vi "Order control references by label order.vi"(8 "error in":errorcluster, 10 "Ordered Labels":string[](array[string]), 11 "Control References":refnum<vi>[](array[refnum])) -> (0 "error out":errorcluster, 3 "Ordered control references":refnum<vi>[](array[refnum]))   [LabVIEW 2017, in "verticalDistribution.lvlib"]
doc: "For a given list of control references, this VI orders the references according to the label array.\n\nEach label that doesn't have a matching control reference is assigned a Not a Refnum value."
uses:
  <vilib>/Utility/vertDist/verticalDistribution.lvlib
panel:
  # "Each label that doesn't \nhave a matching control\nreference will be assigned\na Not a Refnum value."
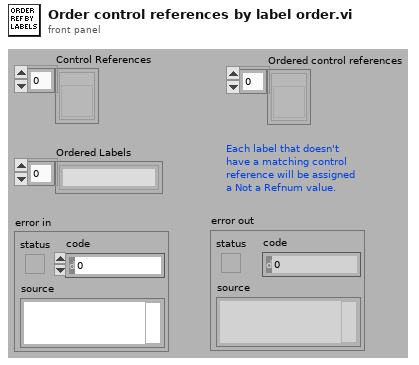
[diagram p1: front panel]
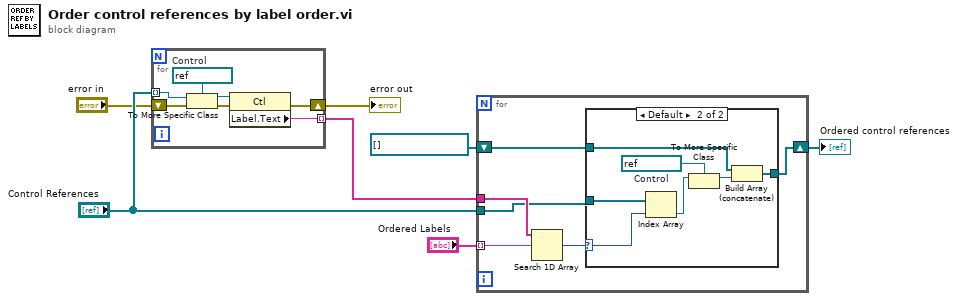
[diagram p0: block diagram]
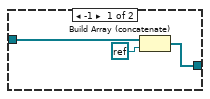
[diagram p2: hidden frame]
diagram:
  n1 = for {
    tunnel: "Control References" -> [w11] mode=indexing
    tunnel: [w9] -> w5 mode=indexing
    shift-right: [w8] -> w2
    shift-left: "error in" -> [w10]
    w12 = refnum<vi> refnum  # Control
    n2 = To More Specific Class(target class=w12, reference=w11, error in=w10) -> (specific class reference=w13:refnum<vi>, error out=w14:errorcluster)
    n3 = property class="Ctl"(reference=w13, error in=w14) -> (error out=w8:errorcluster, "Label.Text"=w9:string)  [unwired: 1 out]
  }
  "error out" <- w2
  n4 = for {
    tunnel: "Ordered Labels" -> [w20] mode=indexing
    tunnel: w5 -> [w19]
    tunnel: "Control References" -> [w16]
    shift-right: [w18] -> w1
    shift-left: refnum<vi>[] [] -> [w17]
    n5 = Search 1D Array(1D array=w19, element=w20) -> (index of element=w15:i32)  [unwired: 1 out]
    n6 = case shown="Default" w15 {
      selector: w15 -> [_ w24]
      tunnel: w16 -> [_ w30]
      tunnel: [w23 w29] -> w18
      tunnel: w17 -> [w21 w28]
      frame -1 {
        n7 = Build Array (concatenate)(w21, refnum<k0> refnum ("Not a Refnum Constant")) -> (w23:refnum<vi>[])
      }
      frame Default {
        w26 = refnum<vi> refnum  # Control
        n8 = Index Array(array=w30, index=w24) -> (element=w27:refnum<vi>)
        n9 = To More Specific Class(target class=w26, reference=w27) -> (specific class reference=w25:refnum<vi>)  [unwired: 1 in, 1 out]
        n10 = Build Array (concatenate)(w28, w25) -> (w29:refnum<vi>[])
      }
    }
  }
  "Ordered control references" <- w1
